vi "TouchTest.vi"() -> ()   [LabVIEW 2025]
uses:
  Controls/Text2Img.ctl
  Controls/TouchXY.ctl
panel:
  out "Image 2":T1(plugin-control)
  in  "Find Font Size":bool
  out "Attempt to Capture":i32[][](array[numeric])
  in  "Size":u16
  in  "Data":string
  out "error out":errorcluster
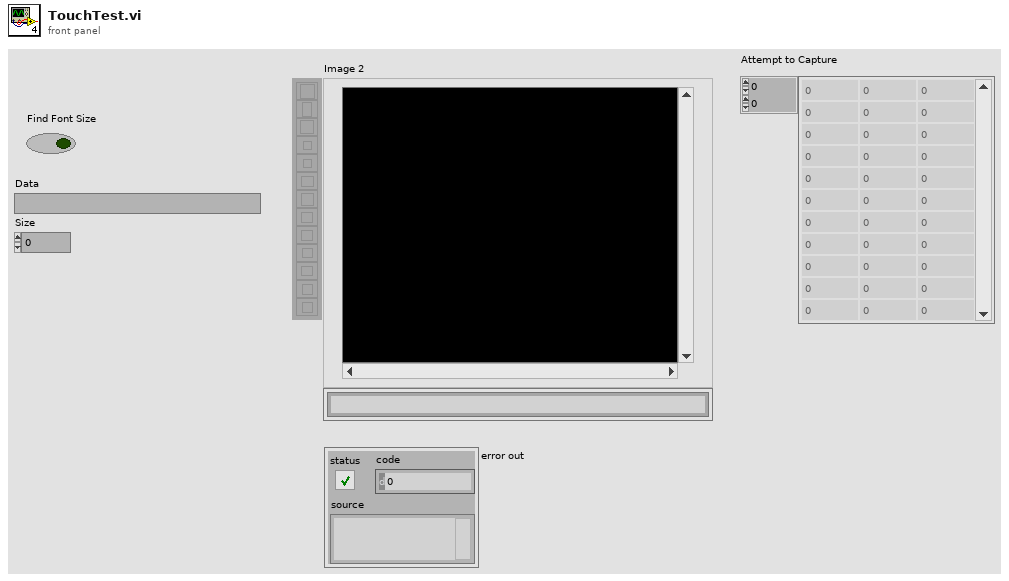
[diagram p1: front panel]
types:
  T1 = typedef "IMAQ Image.ctl" = refnum<image>
  T2 = typedef "Text2Img.ctl" = cluster{"Text.Font":cluster{"Font Name":string, "Size":u16, "Bold":bool, "Italic":bool, "Underline":bool, "Strikeout":bool, "Color":u32}, "Text":string, "Text BG":u32, "Text Color":u32}
  T3 = typedef "IMAQ Rectangle" = cluster{"Left":i32, "Top":i32, "Right":i32, "Bottom":i32, "Rotation":dbl}
  T4 = cluster{"Global Rectangle":i32[], "Contours":cluster{"Contour Type":u32, "ROI Type":u32, "Points":i32[]}[]}
  T5 = typedef "TouchXY.ctl" = cluster{"Win Name":string, "TouchCoord":cluster{"x":sgl, "y":sgl}}
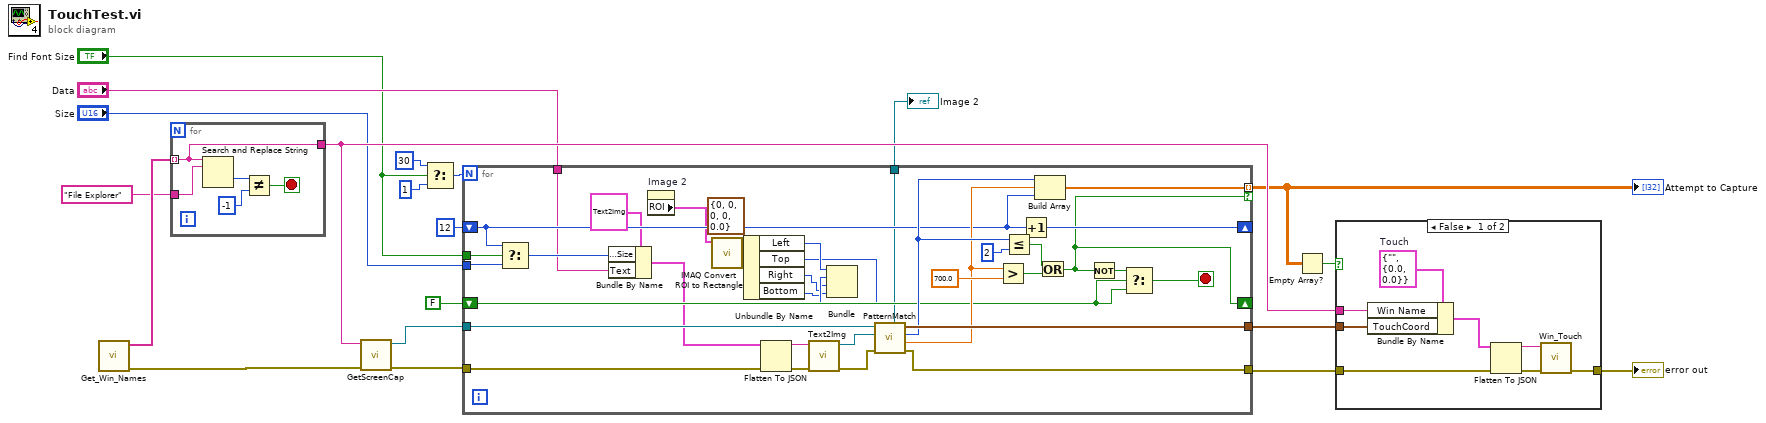
[diagram p0: block diagram]
diagram:
  n1 = call "Get_Win_Names.vi"() -> ("Win_Names"=w19:string[], "error out"=w16:errorcluster)  [unwired: 9 in]
  n2 = for {
    tunnel: w19 -> [w22] mode=indexing
    tunnel: "File Explorer" ("Win Name") -> [w25]
    tunnel: [w22] -> w17
    stop <- w23 stop-if-true
    n3 = Search and Replace String(input string=w22, search string=w25) -> (offset past replacement=w21:i32)  [unwired: 6 in, 3 out]
    n4 = Not Equal?(x=w21, y=-1) -> (x != y?=w23:bool)
  }
  n5 = call "GetScreenCap.vi"("error in (no error)"=w16, "Win Name"=w17) -> ("error out"=w15:errorcluster, "Image Out"=w13:T1)  [unwired: 8 in]
  n6 = Select(t=30 ("f"), s="Find Font Size", f=1) -> (s? t:f=w10:i32)
  n7 = for {
    N: w10 -> [_]
    tunnel: "Data" -> [w36]
    tunnel: w13 -> [w59]
    tunnel: [w55] -> w11
    tunnel: w15 -> [w35]
    tunnel: [w56] -> w12
    tunnel: "Find Font Size" -> [w47]
    tunnel: "Size" -> [w46]
    shift-right: [w54] -> _
    shift-left: u16 12 ("Size") -> [w44]
    tunnel: [w45] -> w1 mode=indexing if=w40
    shift-right: [w40] -> _
    shift-left: FALSE ("x .or. y?") -> [w42]
    tunnel: [w39] -> w3
    stop <- w43 stop-if-true
    (unwired) T3 {"Left"=0, "Top"=0, "Right"=0, "Bottom"=0, "Rotation"=0.0} ("Rectangle")
    n8 = Select(t=w44, s=w47, f=w46) -> (s? t:f=w38:u16)
    n9 = Bundle By Name(cluster=T2 {"Text.Font"={"Font Name"="Segoe UI", "Size"=29, "Bold"=FALSE, "Italic"=FALSE, "Underline"=FALSE, "Strikeout"=FALSE, "Color"=16448250}, "Text"="", "Text BG"=0, "Text Color"=16448250}, "Text.Font.Size"=w38, "Text"=w36) -> (w33:T2)
    n10 = property on="Image 2" class="ImageControl"() -> ("ROI"=w30:T4)  [unwired: 2 in, 2 out]
    n11 = call "IMAQ Convert ROI to Rectangle"("ROI Descriptor"=w30) -> ("Rectangle"=w31:T3)  [unwired: 8 in, 1 out]
    n12 = Unbundle By Name(w31) -> ("Left"=w29:i32, "Top"=w28:i32, "Right"=w27:i32, "Bottom"=w26:i32)
    n13 = Flatten To JSON(anything=w33, error in (no error)=w35) -> (JSON string=w32:string, 11:w34:errorcluster)  [unwired: 1 in]
    n14 = call "Text2Img.vi"("error in (no error)"=w34, "JSON string"=w32) -> ("error out"=w57:errorcluster, "Image"=w58:T1)  [unwired: 8 in]
    n15 = Bundle("Left"=w29, "Top"=w28, "Right"=w27, "Bottom"=w26) -> ()  [unwired: 1 in, 1 out]
    n16 = call "PatternMatch.vi"("error in"=w57, "Template"=w58, "Image"=w59) -> ("error out"=w56:errorcluster, "Score"=w48:sgl, "Attempt"=w53:i32, "Position"=w55:cluster{"x":sgl, "y":sgl}, "Image 2"=w39:T1)  [unwired: 4 in]
    n17 = Greater?(x=w48, y=sgl 700.0) -> (0:w50:bool)
    n18 = Less Or Equal?(x=w53, y=2) -> (x <= y?=w49:bool)
    n19 = Increment(x=w44) -> (x+1=w54:u16)
    n20 = Build Array(w53, w48, w44) -> (w45:sgl[])
    n21 = Or(x=w49, y=w50) -> (x .or. y?=w40:bool)
    n22 = Not(x=w40) -> (.not. x?=w41:bool)
    n23 = Select(t=w41, s=w42, f=w42) -> (s? t:f=w43:bool)
  }
  "Attempt to Capture" <- w1
  "Image 2" <- w3
  n24 = Empty Array?(array=w1) -> (empty?=w2:bool)
  n25 = case shown="False" w2 {
    tunnel: [w67 w68] -> w20
    tunnel: w17 -> [w66 _]
    tunnel: w12 -> [w62 w68]
    tunnel: w11 -> [w65 _]
    frame False {
      w64 = T5 {"Win Name"="", "TouchCoord"={"x"=0.0, "y"=0.0}}  # Touch
      n26 = Bundle By Name(cluster=w64, "Win Name"=w66, "TouchCoord"=w65) -> (w63:T5)
      n27 = Flatten To JSON(anything=w63, error in (no error)=w62) -> (JSON string=w60:string, 11:w61:errorcluster)  [unwired: 1 in]
      n28 = call "Win_Touch.vi"("error in (no error)"=w61, "TouchXY"=w60) -> ("error out"=w67:errorcluster)  [unwired: 9 in]
    }
    frame True {
    }
  }
  "error out" <- w20
